vi "Autonomous Independent.vi"() -> ()   [LabVIEW 2013]
doc: "This VI is called when autonomous begins, and will automatically be terminated when autonomous ends. You can carry out timed or sensor driven robot movement independently without needing to return to the caller."
uses:
  Robot Global Data.vi
  <vilib>/Rock Robotics/WPI/RobotDrive/WPI_RobotDriveGetSetRefNum.vi
  <vilib>/Rock Robotics/WPI/Joystick/WPI_JoystickGetSetRefNum.vi
  <vilib>/Rock Robotics/WPI/RobotDrive/WPI_RobotDriveArcadeDrive_Standard(NoSaturation).vi
panel:
  in  "Autonomous state":enum16{"In firing position", "moving forward"}(ring)
  out "autonomous timer":dbl
  out "Autonomous time elapsed":dbl
  out "Hot?":bool
  out "Current Movement, for debugging":T1 {"Y Joystick Value" scale=1.0..-1.0; "X Joystick Value" scale=-1.0..1.0}
  in  "Array of robot movements":T2(array[cluster]) {"Y Joystick Value" scale=1.0..-1.0; "X Joystick Value" scale=-1.0..1.0}
  # "Be sure to right-click and choose Data Operations>>Make Current Value default if you want to save the array values with the VI"
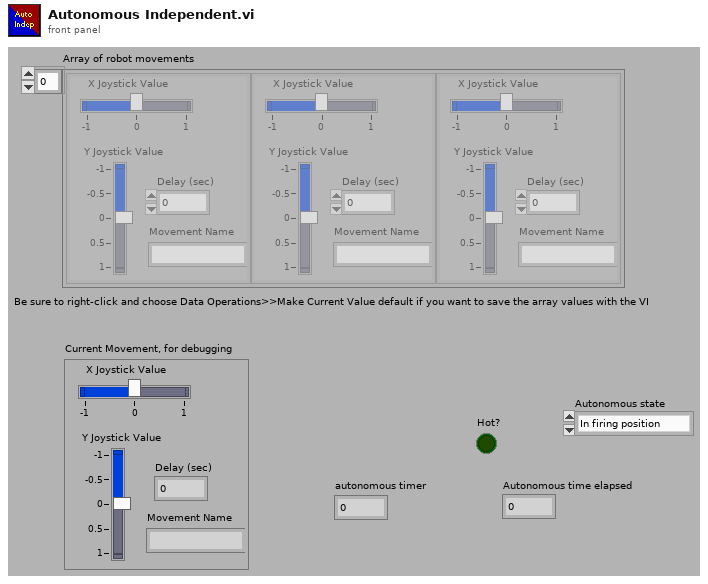
[diagram p1: front panel]
types:
  T1 = cluster{"X Joystick Value":dbl, "Y Joystick Value":dbl, "Delay (sec)":dbl, "Movement Name":string}
  T2 = cluster{"X Joystick Value":dbl, "Y Joystick Value":dbl, "Delay (sec)":dbl, "Movement Name":string}[]
  T3 = typedef "WPI_JoystickDevRef.ctl" = cluster{"Device":T4}
  T4 = typedef "WPI_JoystickDeviceEnum.ctl" = enum16{"USB 1", "USB 2", "USB 3", "USB 4", "Kinect 1", "Kinect 2"}
  T5 = cluster{"axis 1 (x)":dbl, "axis 2 (y)":dbl, "axis 3 (throttle)":dbl, "axis 4":dbl, "axis 5":dbl, "axis 6":dbl}
  T6 = typedef "WPI_EncoderDevRef.ctl" = cluster{"DevStatus":errorcluster, "EncoderIndex":T7, "CounterIndex":T8, "DistancePerCount":dbl, "Decoding Type":T9}
  T7 = typedef "FPGA_EncoderIdx.ctl" = enum8{"Enc 0", "Enc 1", "Enc 2", "Enc 3", "Invalid"}
  T8 = typedef "FPGA_CounterCtrSystemIndex.ctl" = enum8{"Ctr 0", "Ctr 1", "Ctr 2", "Ctr 3", "Ctr 4", "Ctr 5", "Ctr 6", "Ctr 7", "Invalid"}
  T9 = typedef "WPI_EncoderType.ctl" = enum16{"1x", "2x", "4x"}
  T10 = typedef "WPI_RobotDriveDevRef.ctl" = cluster{"DevStatus":errorcluster, "Motors[]":T11[], "Square Inputs":bool, "Max Output":dbl, "Isochronous":bool}
  T11 = typedef "WPI_MotorControlDeviceRef.ctl" = cluster{"DeviceStatus":errorcluster, "Type":enum16{"PWM", "CAN"}, "PWM":cluster{"Digital Module":T12, "PWM Channel":T13, "DeadBand":T14}, "CAN":cluster{"Device Number":u8, "Control Mode":T15, "Semaphore":T16, "Max Vout":dbl}, "Invert":bool, "TransformRef":T17, "InvTransformRef":T17}
  T12 = typedef "FPGA_TypedefDigitalModule.ctl" = enum16{"Digital Module 1", "Digital Module 2"}
  T13 = typedef "FPGA_DIOPWMChannel.ctl" = enum8{"PWM 1", "PWM 2", "PWM 3", "PWM 4", "PWM 5", "PWM 6", "PWM 7", "PWM 8", "PWM 9", "PWM 10", "Invalid"}
  T14 = typedef "WPI_PWMDeadband.ctl" = cluster{"Name":string, "maxPositivePwm":i32, "minPositivePwm":i32, "centerPwm":i32, "maxNegativePwm":i32, "minNegativePwm":i32, "angularRange":u16}
  T15 = typedef "WPI_CANJaguar_ControlMode.ctl" = enum8{"Percent VBus", "Current", "Speed", "Position", "Voltage"}
  T16 = typedef "Semaphore RefNum" = refnum<k1>
  T17 = typedef "WPI_PWMTransform_ConPane.ctl" = refnum<vi>
  T18 = typedef "TargetType.ctl" = enum16{"Not Hot", "Hot"}
  T19 = cluster{"Scores":cluster{"Total":dbl, "Left":dbl, "Right":dbl, "Ratio":dbl, "Vertical":dbl, "index":i32, "State":T18}, "Verticals":cluster{"Horizontal?":bool, "Aspect Score":dbl, "Rect Score":dbl, cluster{"Left":dbl, "Top":dbl, "Right":dbl, "Bottom":dbl}, "Equiv H":dbl, "Equiv V":dbl}, "Horizontals":cluster{"Horizontal?":bool, "Aspect Score":dbl, "Rect Score":dbl, cluster{"Left":dbl, "Top":dbl, "Right":dbl, "Bottom":dbl}, "Equiv H":dbl, "Equiv V":dbl}, "Distance ft":dbl, "Center":cluster{"X":dbl, "Y":dbl}}[]
  T20 = cluster{"Total":dbl, "Left":dbl, "Right":dbl, "Ratio":dbl, "Vertical":dbl, "index":i32, "State":T18}
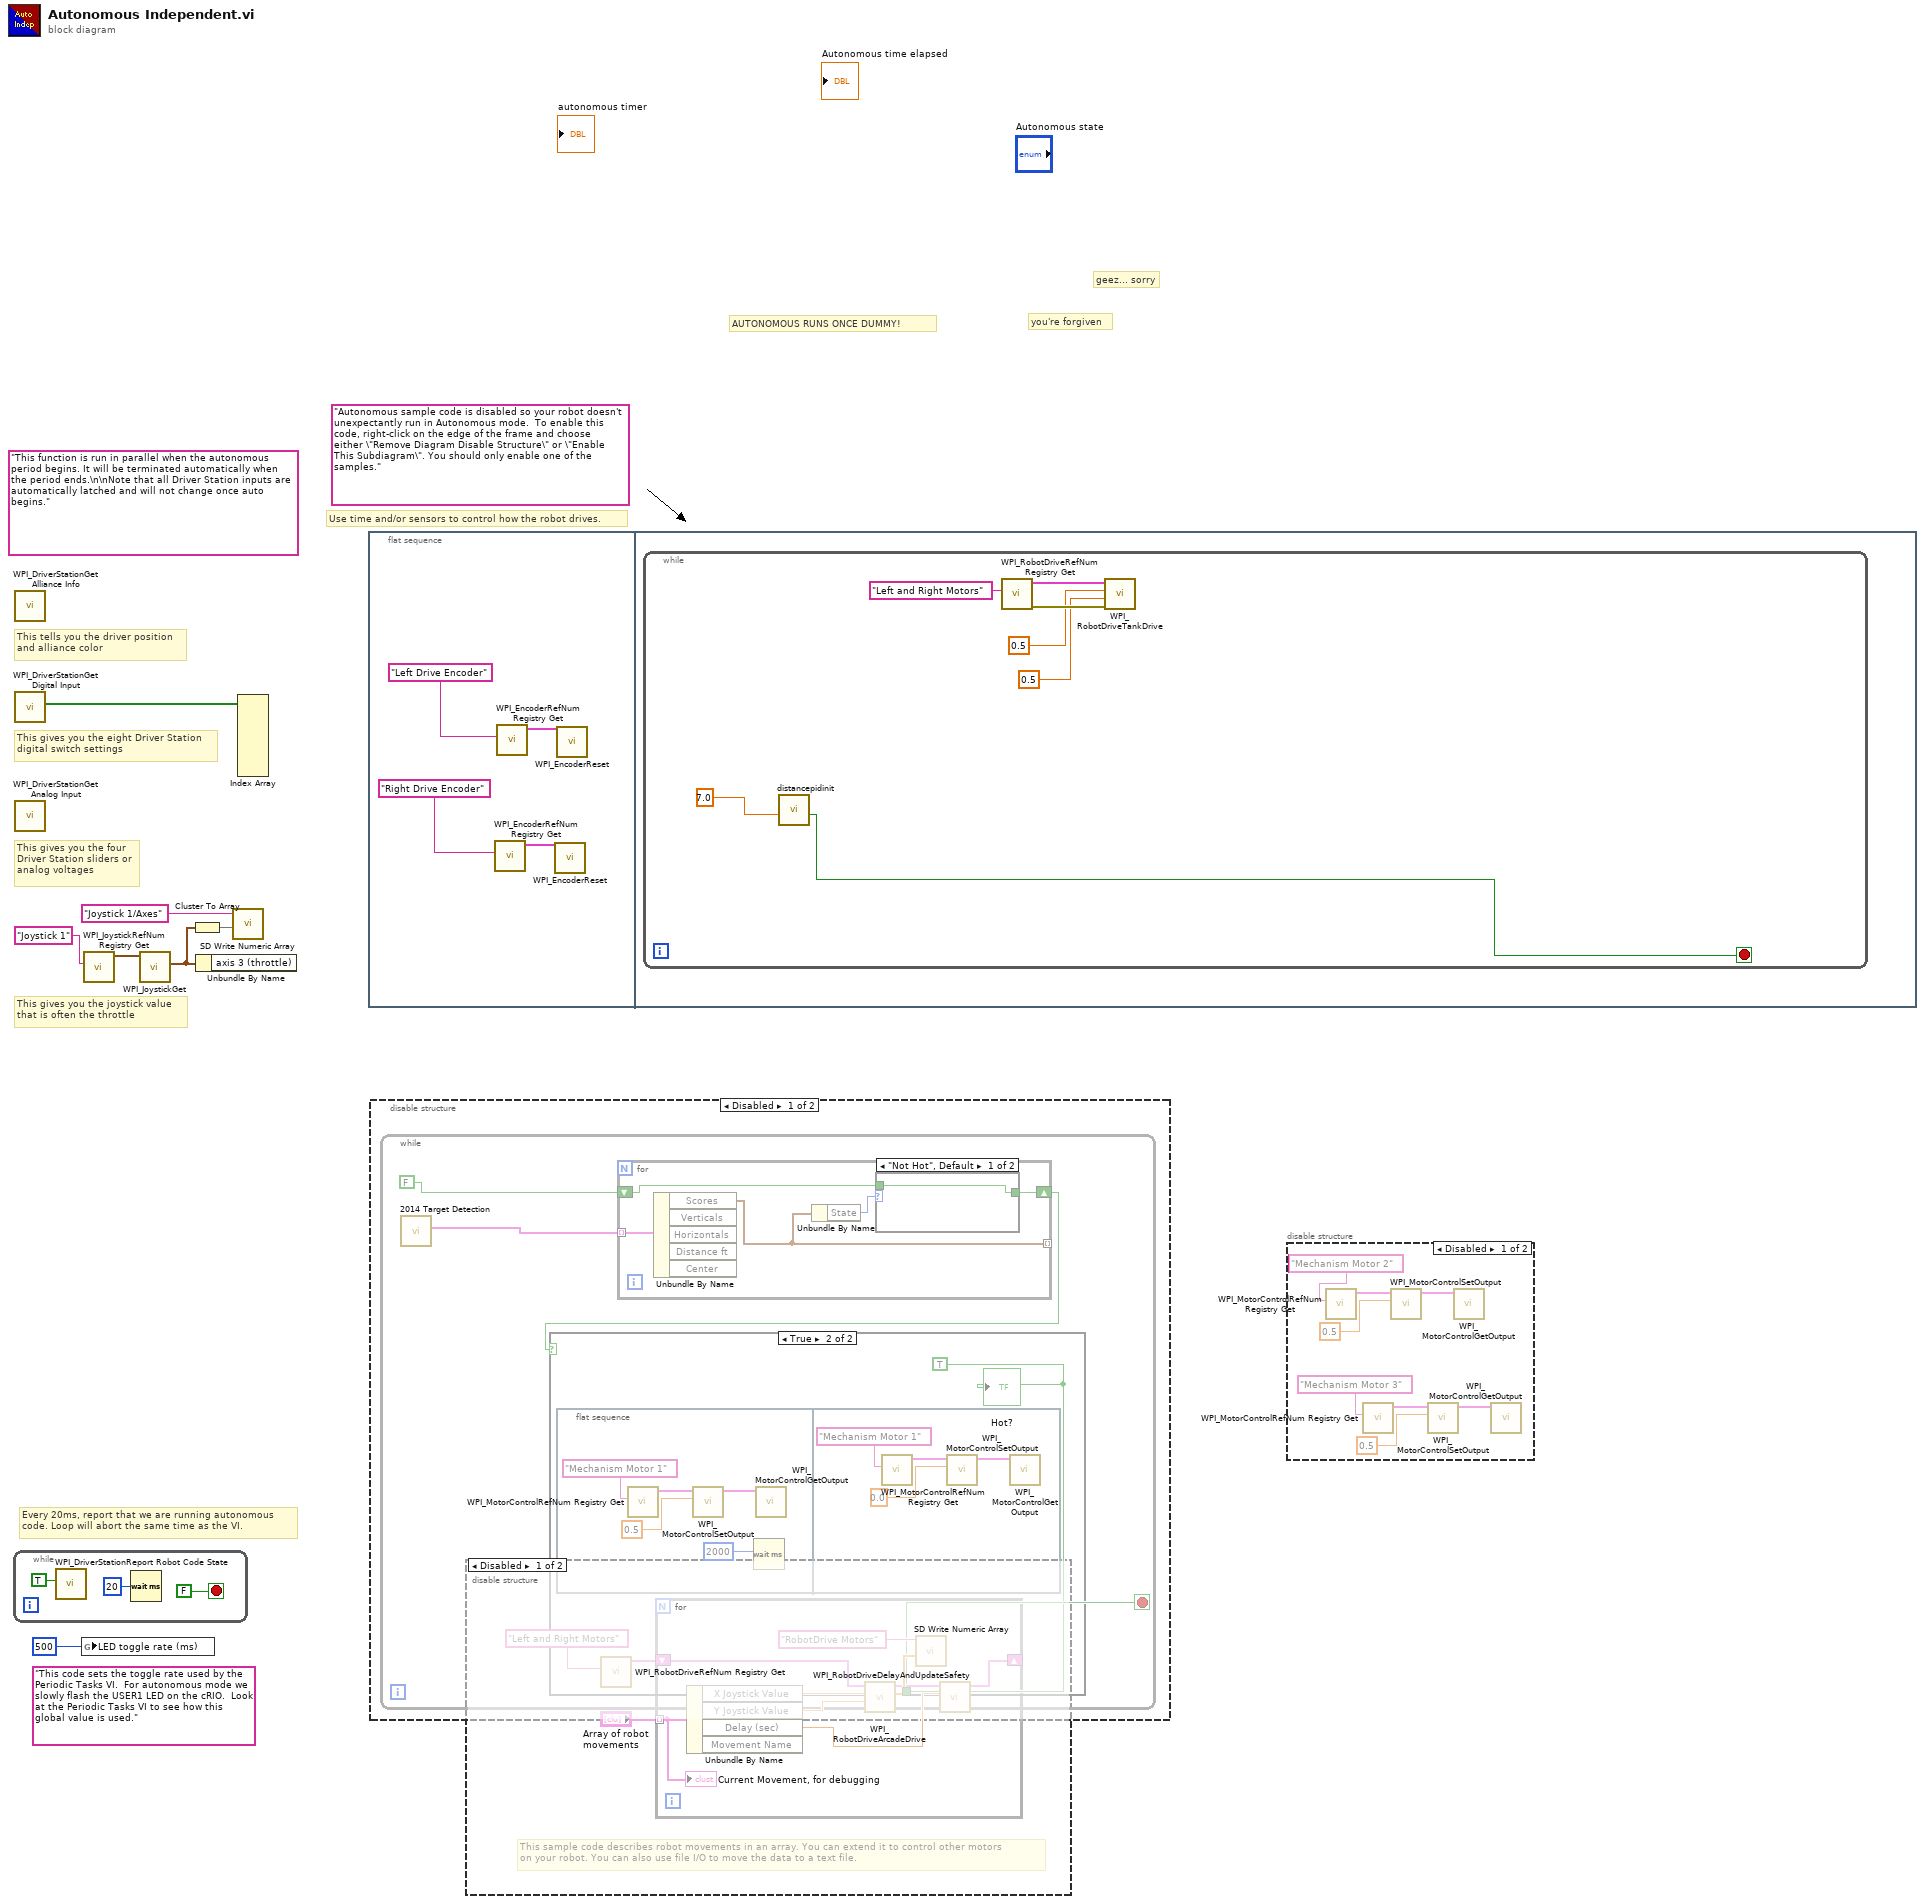
[diagram p0: block diagram]
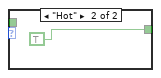
[diagram p2: hidden frame]
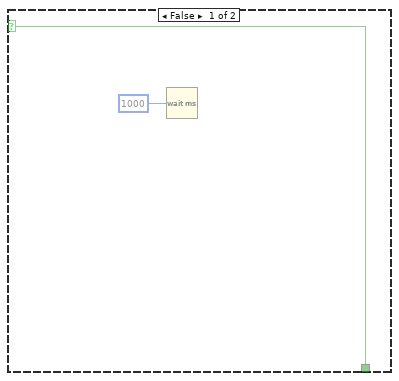
[diagram p3: hidden frame]
diagram:
  (unwired) "This code sets the toggle rate used by the Periodic Tasks VI.  For autonomous mode we slowly flash the USER1 LED on the cRIO.  Look at the Periodic Tasks VI to see how this global value is used."
  (unwired) "Autonomous sample code is disabled so your robot doesn't unexpectantly run in Autonomous mode.  To enable this code, right-click on the edge of the frame and choose either \"Remove Diagram Disable Structure\" or \"Enable This Subdiagram\". You should only enable one of the samples."
  (unwired) "This function is run in parallel when the autonomous period begins. It will be terminated automatically when the period ends.\n\nNote that all Driver Station inputs are automatically latched and will not change once auto begins."
  # "you're forgiven"
  # "geez... sorry"
  # "AUTONOMOUS RUNS ONCE DUMMY!"
  # "Every 20ms, report that we are running autonomous\ncode. Loop will abort the same time as the VI."
  # "This gives you the joystick value\nthat is often the throttle"
  # "Use time and/or sensors to control how the robot drives."
  # "This tells you the driver position\nand alliance color"
  # "This gives you the eight Driver Station\ndigital switch settings"
  # "This gives you the four\nDriver Station sliders or\nanalog voltages"
  n1 = while {
    stop <- FALSE stop-if-true
    n2 = call <vilib>:"WPI_DriverStationReport Robot Code State.vi"("Autonomous"=TRUE) -> ()  [unwired: 10 in, 1 out]
    n3 = Wait (ms)(milliseconds to wait=u32 20) -> ()  [unwired: 1 out]
  }
  n4 = call <vilib>:"WPI_DriverStationGet Alliance Info.vi"() -> ()  [unwired: 12 out]
  n5 = call <vilib>:"WPI_DriverStationGet Digital Input.vi"() -> ("Driver Station Digital Input (1-8)"=w7:bool[])  [unwired: 11 out]
  n6 = call <vilib>:"WPI_DriverStationGet Analog Input.vi"() -> ()  [unwired: 12 out]
  n7 = global write "Robot Global Data.vi" "LED toggle rate (ms)"(u32 500 ("LED ms toggle rate")) -> ()
  n8 = call <vilib>:"WPI_JoystickRefNum Registry Get.vi"("refnum name"="Joystick 1") -> ("JoystickDevRef"=w5:T3)  [unwired: 1 in, 9 out]
  n9 = call <vilib>:"WPI_JoystickGet.vi"("JoystickDevRef"=w5) -> ("Axes"=w2:T5)  [unwired: 1 in, 5 out]
  n10 = Cluster To Array(cluster=w2) -> (array=w3:dbl[])
  n11 = Unbundle By Name(w2) -> ()  [unwired: 1 out]
  n12 = call <vilib>:"SD Write Numeric Array.vi"("Numeric Array"=w3, "Name"="Joystick 1/Axes") -> ()  [unwired: 8 in, 2 out]
  n13 = Index Array(array=w7) -> ()  [unwired: 8 in, 8 out]
  n14 = flat-sequence {
    frame #0 {
      n15 = call <vilib>:"WPI_EncoderRefNum Registry Get.vi"("refnum name"="Right Drive Encoder") -> ("EncoderDevRef"=w11:T6)  [unwired: 9 in, 1 out]
      n16 = call <vilib>:"WPI_EncoderRefNum Registry Get.vi"("refnum name"="Left Drive Encoder") -> ("EncoderDevRef"=w13:T6)  [unwired: 9 in, 1 out]
      n17 = call <vilib>:"WPI_EncoderReset.vi"("EncoderDevRef"=w11) -> ()  [unwired: 9 in, 2 out]
      n18 = call <vilib>:"WPI_EncoderReset.vi"("EncoderDevRef"=w13) -> ()  [unwired: 9 in, 2 out]
    }
    frame #1 {
      n19 = while {
        stop <- w17 stop-if-true
        n20 = call "distancepidinit.vi"("Distance From Target"=7.0) -> ("Done?"=w17:bool)  [unwired: 10 in]
        n21 = call <vilib>:"WPI_RobotDriveRefNum Registry Get.vi"("refnum name"="Left and Right Motors") -> ("error out"=w20:errorcluster, "RobotDriveDevRef"=w21:T10)  [unwired: 9 in]
        n22 = call <vilib>:"WPI_RobotDriveTankDrive.vi"("error in (no error)"=w20, "Right axis value"=0.5, "Left axis value"=0.5, "RobotDriveDevRef"=w21) -> ()  [unwired: 5 in, 3 out]
      }
    }
  }
  n23 = disable-structure shown="Disabled" {
    frame Disabled {
      n24 = while {
        stop <- w25 stop-if-true
        n25 = call "2014 Target Detection.vi"() -> ("Target Info"=w24:T19)  [unwired: 11 in]
        n26 = for {
          tunnel: w24 -> [w30] mode=indexing
          tunnel: [w29] -> _ mode=indexing
          shift-right: [w27] -> w22
          shift-left: FALSE -> [w26]
          n27 = Unbundle By Name(w30) -> ("Scores"=w29:T20)  [unwired: 4 out]
          n28 = Unbundle By Name(w29) -> ("State"=w28:T18)
          n29 = case shown="\"Not Hot\", Default" w28 {
            tunnel: [w31 TRUE] -> w27
            tunnel: w26 -> [w31 _]
            frame "Not Hot", Default {
            }
            frame "Hot" {
            }
          }
        }
        n30 = case shown="True" w22 {
          selector: w22 -> [w33 _]
          tunnel: [w33 w35] -> w25
          frame False {
            n31 = Wait (ms)(milliseconds to wait=1000) -> ()  [unwired: 1 out]
          }
          frame True {
            w35 = TRUE
            n32 = flat-sequence {
              frame #0 {
                n33 = call <vilib>:"WPI_MotorControlRefNum Registry Get.vi"("refnum name"="Mechanism Motor 1") -> ("MotorControlDevRef"=w39:T11)  [unwired: 9 in, 1 out]
                n34 = call <vilib>:"WPI_MotorControlSetOutput.vi"("Output"=0.5, "MotorControlDevRef"=w39) -> ("MotorControlDevRef"=w37:T11)  [unwired: 7 in, 2 out]
                n35 = Wait (ms)(milliseconds to wait=2000) -> ()  [unwired: 1 out]
                n36 = call <vilib>:"WPI_MotorControlGetOutput.vi"("MotorControlDevRef"=w37) -> ()  [unwired: 8 in, 3 out]
              }
              frame #1 {
                n37 = call <vilib>:"WPI_MotorControlRefNum Registry Get.vi"("refnum name"="Mechanism Motor 1") -> ("MotorControlDevRef"=w43:T11)  [unwired: 9 in, 1 out]
                n38 = call <vilib>:"WPI_MotorControlSetOutput.vi"("Output"=0.0, "MotorControlDevRef"=w43) -> ("MotorControlDevRef"=w41:T11)  [unwired: 7 in, 2 out]
                n39 = call <vilib>:"WPI_MotorControlGetOutput.vi"("MotorControlDevRef"=w41) -> ()  [unwired: 8 in, 3 out]
              }
            }
            "Hot?" <- w35
          }
        }
      }
    }
    frame Enabled {
    }
  }
  n40 = disable-structure shown="Disabled" {
    frame Disabled {
      # "This sample code describes robot movements in an array. You can extend it to control other motors\non your robot. You can also use file I/O to move the data to a text file."
      n41 = call <vilib>:"WPI_RobotDriveRefNum Registry Get.vi"("refnum name"="Left and Right Motors") -> ("RobotDriveDevRef"=w46:T10)  [unwired: 1 in, 9 out]
      n42 = for {
        shift-right: [w52] -> _
        shift-left: w46 -> [w53]
        tunnel: "Array of robot movements" -> [w48] mode=indexing
        n43 = Unbundle By Name(w48) -> ("X Joystick Value"=w51:dbl, "Y Joystick Value"=w50:dbl, "Delay (sec)"=w49:dbl)  [unwired: 1 out]
        n44 = call-poly <vilib>:"WPI_RobotDriveArcadeDrive.vi"("Y axis value"=w50, "X axis value"=w51, "RobotDriveDevRef"=w53) -> ("Motor Values"=w55:dbl[], "RobotDriveDevRef"=w54:T10)  [unwired: 1 in, 6 out]
        n45 = call <vilib>:"SD Write Numeric Array.vi"("Numeric Array"=w55, "Name"="RobotDrive Motors") -> ()  [unwired: 8 in, 2 out]
        n46 = call <vilib>:"WPI_RobotDriveDelayAndUpdateSafety.vi"("Delay (s)"=w49, "RobotDriveDevRef"=w54) -> ("RobotDriveDevRef 2"=w52:T10)  [unwired: 8 in, 1 out]
        "Current Movement, for debugging" <- w48
      }
    }
    frame Enabled {
    }
  }
  n47 = disable-structure shown="Disabled" {
    frame Disabled {
      n48 = call <vilib>:"WPI_MotorControlRefNum Registry Get.vi"("refnum name"="Mechanism Motor 2") -> ("MotorControlDevRef"=w64:T11)  [unwired: 9 in, 1 out]
      n49 = call <vilib>:"WPI_MotorControlRefNum Registry Get.vi"("refnum name"="Mechanism Motor 3") -> ("MotorControlDevRef"=w59:T11)  [unwired: 9 in, 1 out]
      n50 = call <vilib>:"WPI_MotorControlSetOutput.vi"("Output"=0.5, "MotorControlDevRef"=w64) -> ("MotorControlDevRef"=w62:T11)  [unwired: 7 in, 2 out]
      n51 = call <vilib>:"WPI_MotorControlSetOutput.vi"("Output"=0.5, "MotorControlDevRef"=w59) -> ("MotorControlDevRef"=w57:T11)  [unwired: 7 in, 2 out]
      n52 = call <vilib>:"WPI_MotorControlGetOutput.vi"("MotorControlDevRef"=w62) -> ()  [unwired: 8 in, 3 out]
      n53 = call <vilib>:"WPI_MotorControlGetOutput.vi"("MotorControlDevRef"=w57) -> ()  [unwired: 8 in, 3 out]
    }
    frame Enabled {
    }
  }
